vi "[EIP型数字化反应性仪ETH].vi"() -> ()   [LabVIEW 2020]
doc: "该范例演示了通过VI查看其它VI的方法，还可运行和中止查看的VI。\n对于要中止的VI，应设置为可中止。对于无法中止的VI，可查看相关范例。"
uses:
  <vilib>/Utility/error.llb/DialogType.ctl
  GlobalVariable.vi
  TCPModbus_MasterClient/MB Ethernet Master Query Write Multiple Registers (poly).vi
  TCPModbus_MasterClient/MB Ethernet Master Query Read Input Registers (poly).vi
  <vilib>/Analysis/polynomials.llb/Scalar Polynomial Evaluation (DBL).vi
  <vilib>/Analysis/NI_AALPro.lvlib
panel:
  out "上段":bool
  out "下段":bool
  in  "修正因子文件状态":bool
  in  "周期拟合与反应性":bool
  in  "多通道并行实测":bool
  in  "物理参数设置":bool
  in  "打开文件夹":bool
  in  "返回LOGO":bool
  out "项名称":string
  out "退出":bool
  out "MainPanel":enum32{"panel", "logo"}(tab)=enum."logo"
  in  "校准时间":bool
  in  "更新物理参数":bool
  in  "高压2":dbl(slide) scale=-500.0..500.0
  in  "高压1":dbl(slide) scale=-500.0..500.0
  out "P2_8":dbl format="%#.4g"
  out "P2_7":dbl format="%#.4g"
  out "P2_6":dbl format="%#.4g"
  out "P2_5":dbl format="%#.4g"
  out "P2_4":dbl format="%#.4g"
  out "P2_3":dbl format="%#.4g"
  out "P2_1":dbl format="%#.4g"
  in  "离线数据源":bool
  out "电脑历时":dbl format="%#.2g"
  out "程序历时":dbl format="%#.2g"
  out "累计时差":dbl format="%#.4f"
  out "脉冲2":dbl(knob) scale=1.0..1000000.0 scale format="%#_3g"
  out "脉冲3":dbl(knob) scale=1.0..1000000.0 scale format="%#_3g"
  out "电流1":dbl(slide) scale=1e-13..0.0001 scale format="%#_2e"
  out "电流2":dbl(slide) scale=1e-13..0.0001 scale format="%#_2e"
  out "电压1":dbl(knob) scale=1.0..5.0 scale format="%#.4f"
  out "电压2":dbl(knob) scale=1.0..5.0 scale format="%#.4f"
  out "电压3":dbl(knob) scale=1.0..5.0 scale format="%#.4f"
  out "电压4":dbl(knob) scale=1.0..5.0 scale format="%#.4f"
  out "电压5":dbl(knob) scale=1.0..5.0 scale format="%#.4f"
  out "电压6":dbl(knob) scale=1.0..5.0 scale format="%#.4f"
  out "电压7":dbl(knob) scale=1.0..5.0 scale format="%#.4f"
  out "电压8":dbl(knob) scale=1.0..5.0 scale format="%#.4f"
  out "脉冲1":dbl(knob) scale=1.0..1000000.0 scale format="%#_3g"
  out "P2_2":dbl format="%#.4g"
  # "Current1"
  # "Current2"
  # "NetWork"
  # "Voltage Output"
  # "Voltage Input"
  # "AC220V"
  # "Pulse2"
  # "Pulse3"
  # "GND"
  # "Pulse1"
  # "HV1"
  # "HV2"
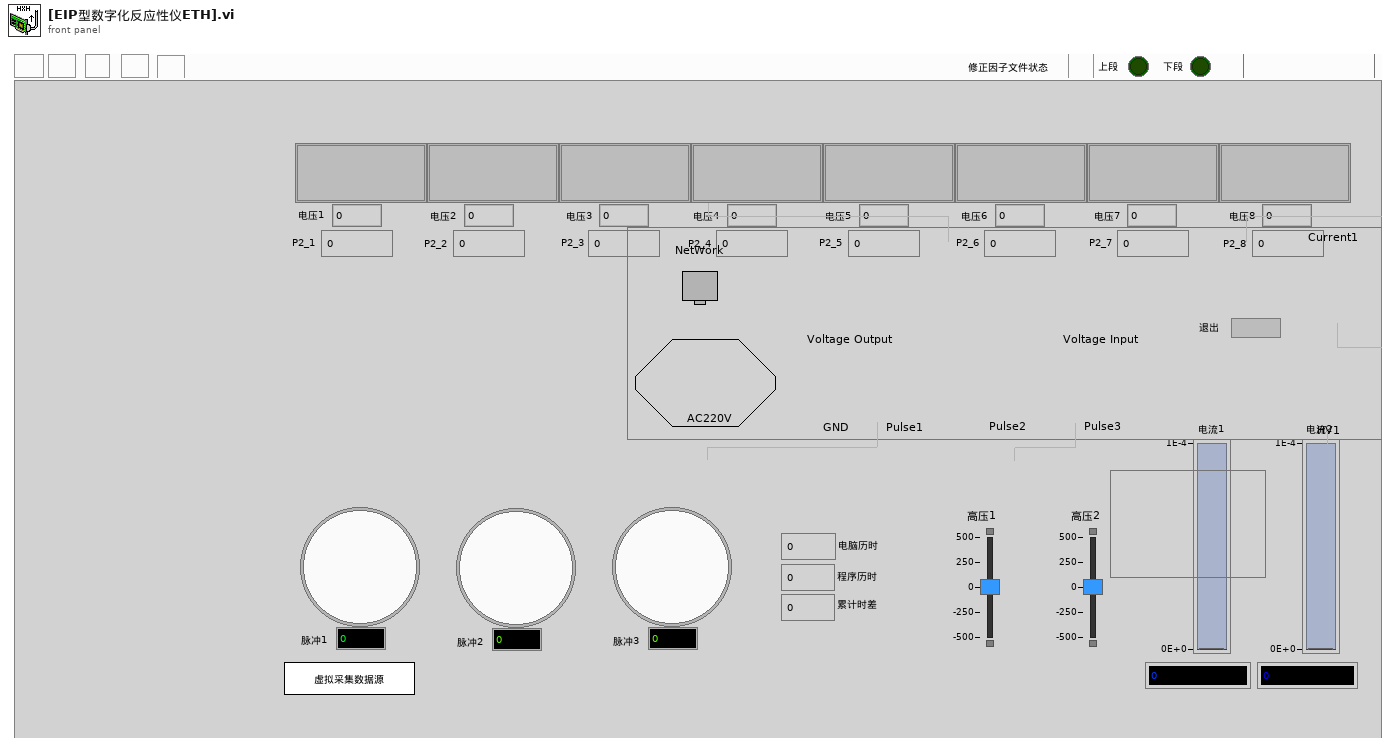
[diagram p1: front panel]
types:
  T1 = typedef "DialogType.ctl" = u16
  T2 = enum32{"Invalid", "Standard", "Closed", "Hidden", "Minimized", "Maximized"}
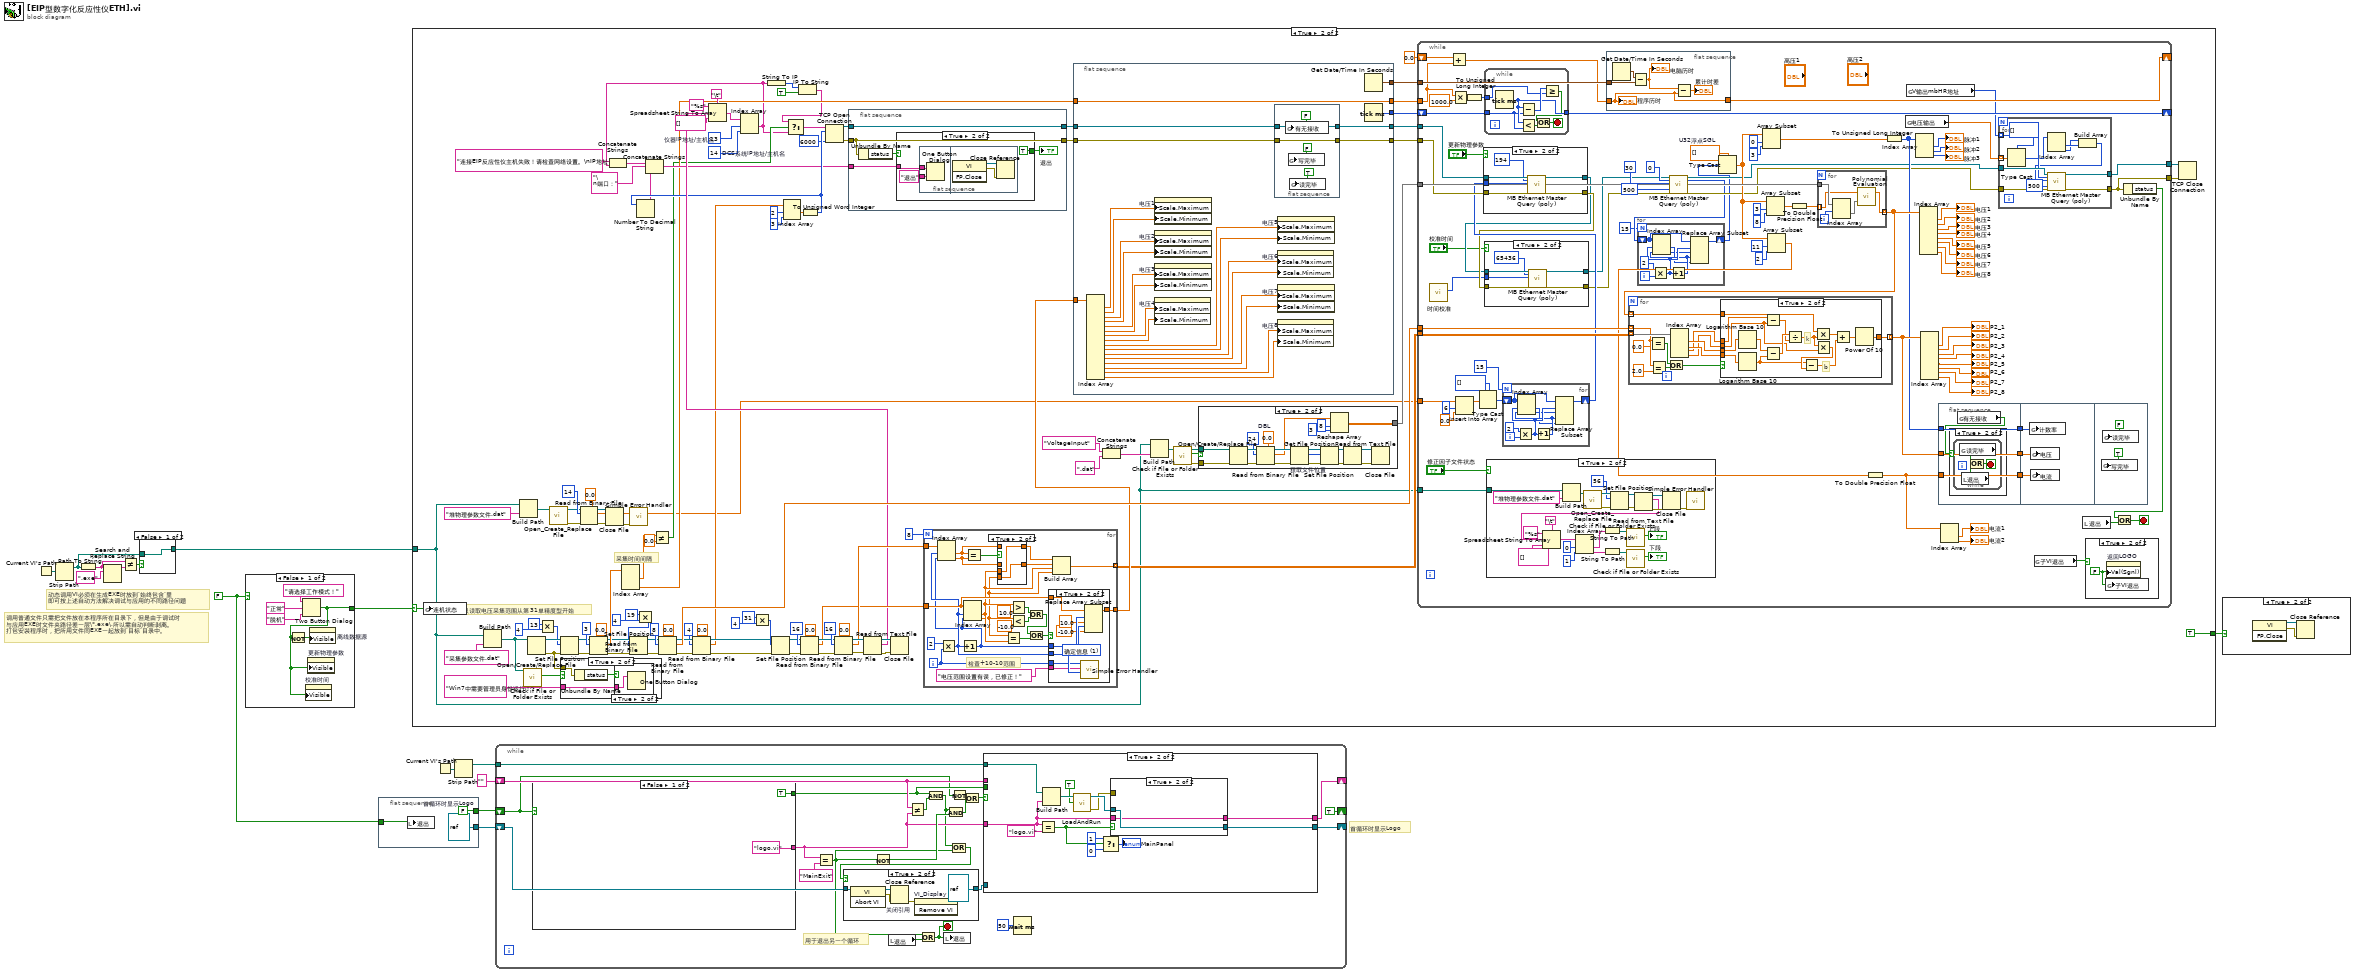
[diagram p0: block diagram]
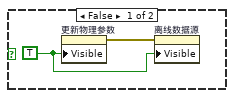
[diagram p2: hidden frame]
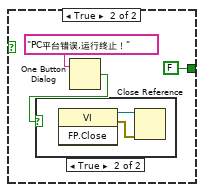
[diagram p3: hidden frame]
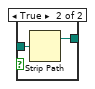
[diagram p5: hidden frame]
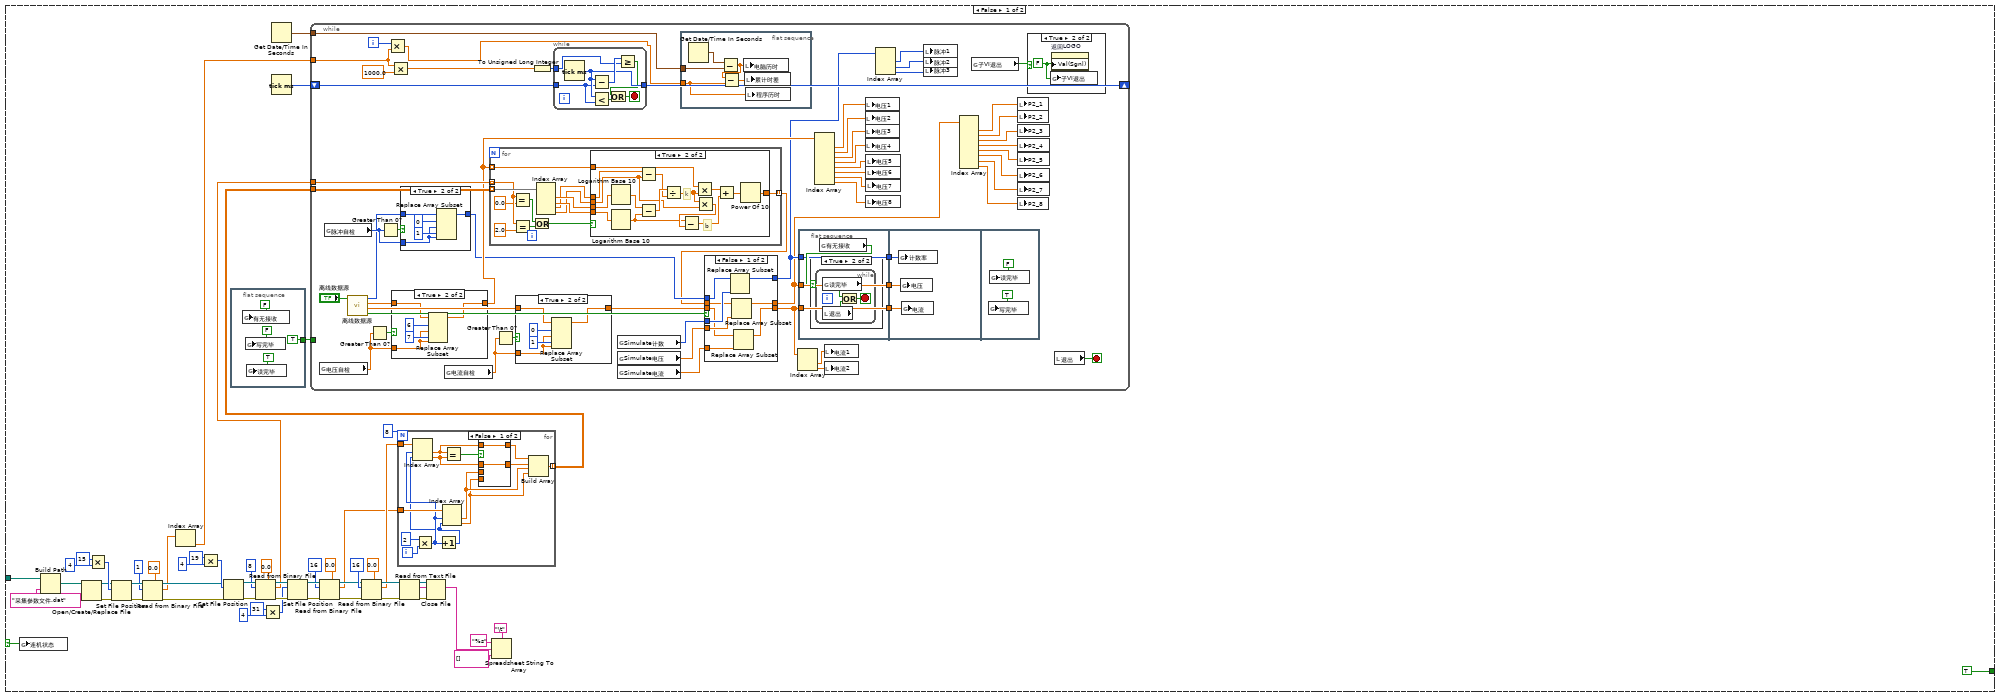
[diagram p6: hidden frame]
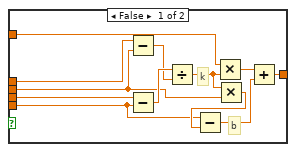
[diagram p12: hidden frame]
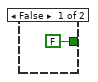
[diagram p15: hidden frame]
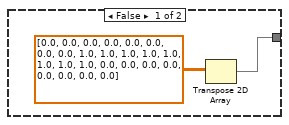
[diagram p18: hidden frame]
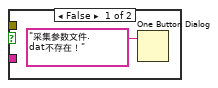
[diagram p19: hidden frame]
diagram:
  w1 = FALSE
  # "调用普通文件只需把文件放在本程序所在目录下，但是由于调试时\n与应用EXE时文件夹路径差一层\\*.exe\\,所以需自动判断剥离。\n打包安装程序时，把所用文件同EXE一起放到‘目标’目录中。"
  # "动态调用VI必须在生成EXE时放到‘始终包含’里\n即可按上述自动方法解决调试与应用的不同路径问题"
  # "首循环时显示Logo"
  n1 = Current VI's Path() -> (path=w10:path)
  n2 = Strip Path(path=w10) -> (stripped path=w5:path)  [unwired: 1 out]
  n3 = Path To String(path=w5) -> (string=w7:string)
  n4 = Search and Replace String(input string=w7, search string=".exe" ("搜索字符串")) -> (result string=w8:string)  [unwired: 6 in, 3 out]
  n5 = Not Equal?(x=w7, y=w8) -> (x != y?=w6:bool)
  n6 = case shown="False" w6 {
    tunnel: w5 -> [w16 w18]
    tunnel: [w16 w17] -> w2
    frame False {
    }
    frame True {
      n7 = Strip Path(path=w18) -> (stripped path=w17:path)  [unwired: 1 out]
    }
  }
  n8 = case shown="False" w1 {
    tunnel: [w19 FALSE ("T button?")] -> w4
    frame False {
      n9 = Two Button Dialog(message="请选择工作模式！" ("消息"), 1:"脱机" ("F按钮名称（“取消”）"), 2:"正常" ("T按钮名称（“确定”）")) -> (T button?=w19:bool)
      n10 = Not(x=w19) -> (.not. x?=w20:bool)
      n11 = property on="校准时间" class="Bool"("Visible"=w19) -> ()  [unwired: 2 in, 2 out]
      n12 = property on="更新物理参数" class="Bool"("Visible"=w19) -> ()  [unwired: 2 in, 2 out]
      n13 = property on="离线数据源" class="Bool"("Visible"=w20) -> ()  [unwired: 2 in, 2 out]
    }
    frame True {
      n14 = One Button Dialog(message="PC平台错误,运行终止！" ("消息")) -> (true=w24:bool)  [unwired: 1 in]
      n15 = case shown="True" w24 {
        frame False {
        }
        frame True {
          n16 = invoke class="VI" method="FP.Close"() -> (reference out=w27:refnum<vi>, error out=w28:errorcluster)  [unwired: 3 in, 1 out]
          n17 = Close Reference(reference=w27, error in (no error)=w28) -> ()  [unwired: 1 out]
        }
      }
    }
  }
  n18 = flat-sequence {
    tunnel: [refnum<vi> refnum ("VI Ref")] -> w15
    tunnel: [w30] -> w14
    tunnel: w1 -> [w29]
    frame #0 {
      w30 = FALSE  # 首循环时显示Logo
      n19 = local write "退出"(w29) -> ()
    }
  }
  n20 = case shown="True" w4 {
    selector: w4 -> [w34 w272]
    tunnel: w2 -> [w64 w266]
    tunnel: [TRUE ("首循环时显示Logo") TRUE ("首循环时显示Logo")] -> w3
    frame False {
      n21 = global write "GlobalVariable.vi" "连机状态"(w34) -> ()
      n22 = Build Path(base path=w64, name or relative path="采集参数文件.dat") -> (appended path=w66:path)
      n23 = Open/Create/Replace File(file path (use dialog)=w66) -> (refnum out=w54:refnum<file>, error out=w53:errorcluster)  [unwired: 5 in, 1 out]
      n24 = Multiply(x=i64 15 ("偏移量（字节）（0）"), y=i64 4 ("偏移量（字节）（0）")) -> (x*y=w61:i64)
      n25 = Set File Position(offset (in bytes) (0)=w61, refnum=w54, error in=w53) -> (refnum out=w57:refnum<file>, error out=w58:errorcluster)  [unwired: 1 in]
      n26 = Read from Binary File(5:sgl 0.0 ("byte stream type"), 8:w58, 10:1 ("count"), 11:w57) -> (0:w51:errorcluster, 2:w50:sgl[], 3:w52:refnum<file>)  [unwired: 2 in, 1 out]
      n27 = Index Array(array=w50) -> (element=w49:sgl)  [unwired: 1 in]
      n28 = Multiply(x=i64 19 ("偏移量（字节）（0）"), y=i64 4 ("偏移量（字节）（0）")) -> (x*y=w73:i64)
      n29 = Set File Position(offset (in bytes) (0)=w73, refnum=w52, error in=w51) -> (refnum out=w69:refnum<file>, error out=w70:errorcluster)  [unwired: 1 in]
      n30 = flat-sequence {
        tunnel: [TRUE ("读完毕")] -> w85
        frame #0 {
          n31 = global write "GlobalVariable.vi" "有无接收"(FALSE ("读完毕")) -> ()
          n32 = global write "GlobalVariable.vi" "写完毕"(FALSE ("读完毕")) -> ()
          n33 = global write "GlobalVariable.vi" "读完毕"(TRUE ("读完毕")) -> ()
        }
      }
      n34 = Read from Binary File(5:sgl 0.0 ("byte stream type"), 8:w70, 10:8 ("count"), 11:w69) -> (0:w81:errorcluster, 2:w63:sgl[], 3:w80:refnum<file>)  [unwired: 2 in, 1 out]
      n35 = Multiply(x=i64 31 ("偏移量（字节）（0）"), y=i64 4 ("偏移量（字节）（0）")) -> (x*y=w79:i64)
      n36 = Get Date/Time In Seconds() -> (seconds since 1Jan1904=w33:timestamp)
      n37 = Tick Count (ms)() -> (millisecond timer value=w32:u32)
      n38 = Set File Position(offset (in bytes) (0)=w79, refnum=w80, error in=w81) -> (refnum out=w76:refnum<file>, error out=w77:errorcluster)  [unwired: 1 in]
      n39 = Read from Binary File(5:sgl 0.0 ("byte stream type"), 8:w77, 10:16 ("count"), 11:w76) -> (0:w45:errorcluster, 2:w40:sgl[], 3:w46:refnum<file>)  [unwired: 2 in, 1 out]
      n40 = Read from Binary File(5:sgl 0.0 ("byte stream type"), 8:w45, 10:16 ("count"), 11:w46) -> (0:w43:errorcluster, 2:w41:sgl[], 3:w44:refnum<file>)  [unwired: 2 in, 1 out]
      n41 = for {
        N: 8 -> [_]
        tunnel: w40 -> [w98]
        tunnel: [w87] -> w39 mode=indexing
        tunnel: w41 -> [w86]
        i -> [w97]
        n42 = Multiply(x=2, y=w97) -> (x*y=w95:i32)
        n43 = Increment(x=w95) -> (x+1=w94:i32)
        n44 = Index Array(array=w86, index #1=w95, index #2=w94) -> (element #1=w93:sgl, element #2=w92:sgl)
        n45 = Index Array(array=w98, index #1=w95, index #2=w94) -> (element #1=w89:sgl, element #2=w88:sgl)
        n46 = Equal?(x=w93, y=w92) -> (x = y?=w96:bool)
        n47 = case shown="False" w96 {
          tunnel: w89 -> [_ w103]
          tunnel: w88 -> [_ w102]
          tunnel: [w101 w103] -> w91
          tunnel: w93 -> [w101 _]
          tunnel: w92 -> [w100 _]
          tunnel: [w100 w102] -> w90
          frame False {
          }
          frame True {
          }
        }
        n48 = Build Array(w91, w90, w89, w88) -> (w87:sgl[])
      }
      n49 = while {
        tunnel: w85 -> [_]
        tunnel: w63 -> [w158]
        tunnel: w49 -> [w135]
        tunnel: w39 -> [w159]
        tunnel: w33 -> [w131]
        shift-right: [w129] -> _
        shift-left: w32 -> [w132]
        i -> [w144]
        stop <- w162 stop-if-true
        n50 = global read "GlobalVariable.vi" "电压自检"() -> (w140:dbl)
        n51 = global read "GlobalVariable.vi" "脉冲自检"() -> (w138:i32)
        n52 = call "离线数据源.vi"("显示前面板"="离线数据源") -> ("前面板打开"=w125:bool, "电流"=w122:dbl[], "电压数据"=w123:dbl[], "脉冲数据"=w124:u32[])  [unwired: 7 in]
        n53 = Greater Than 0?(x=w140) -> (x > 0?=w141:bool)
        n54 = Greater Than 0?(x=w138) -> (x > 0?=w137:bool)
        n55 = Multiply(x=w144, y=w135) -> (x*y=w130:sgl)
        n56 = Multiply(x=w135, y=sgl 1000.0) -> (x*y=w133:sgl)
        n57 = case shown="True" w141 {
          tunnel: w123 -> [w196 w201]
          tunnel: [w196 w200] -> w139
          tunnel: w140 -> [_ w197]
          frame False {
          }
          frame True {
            n58 = Replace Array Subset(array=w201, new element #1=w197, index #1=6 ("索引"), new element #2=w197, index #2=7 ("索引")) -> (w200:dbl[])
          }
        }
        n59 = case shown="True" w137 {
          tunnel: w124 -> [w190 w195]
          tunnel: [w190 w194] -> w119
          tunnel: w138 -> [_ w191]
          frame False {
          }
          frame True {
            n60 = Replace Array Subset(array=w195, new element #1=w191, index #1=0 ("索引"), new element #2=w191, index #2=1 ("索引")) -> (w194:u32[])
          }
        }
        n61 = global read "GlobalVariable.vi" "电流自检"() -> (w142:dbl)
        n62 = for {
          tunnel: w139 -> [w219] mode=indexing
          tunnel: [w208] -> w115 mode=indexing
          tunnel: w159 -> [w220] mode=indexing
          tunnel: w158 -> [w218] mode=indexing
          n63 = Equal?(x=w218, y=sgl 0.0) -> (x = y?=w215:bool)
          n64 = Equal?(x=w218, y=sgl 2.0) -> (x = y?=w214:bool)
          n65 = Or(x=w215, y=w214) -> (x .or. y?=w213:bool)
          n66 = Index Array(array=w220) -> (element #1=w212:sgl, element #2=w211:sgl, element #3=w210:sgl, element #4=w209:sgl)  [unwired: 4 in]
          n67 = case shown="True" w213 {
            tunnel: w219 -> [w232 w238]
            tunnel: [w231 w236] -> w208
            tunnel: w210 -> [w224 w241]
            tunnel: w209 -> [w223 w240]
            tunnel: w212 -> [w222 w234]
            tunnel: w211 -> [w221 w239]
            frame False {
              # "b"
              # "k"
              n68 = Subtract(x=w224, y=w223) -> (x-y=w229:sgl)
              n69 = Subtract(x=w222, y=w221) -> (x-y=w230:sgl)
              n70 = Divide(x=w230, y=w229) -> (x/y=w228:sgl)
              n71 = Multiply(x=w232, y=w228) -> (x*y=w226:dbl)
              n72 = Multiply(x=w228, y=w223) -> (x*y=w227:sgl)
              n73 = Subtract(x=w221, y=w227) -> (x-y=w225:sgl)
              n74 = Add(x=w226, y=w225) -> (x+y=w231:dbl)
            }
            frame True {
              # "b"
              # "k"
              n75 = Logarithm Base 10(1:w234) -> (0:w233:sgl)
              n76 = Logarithm Base 10(1:w239) -> (0:w235:sgl)
              n77 = Subtract(x=w241, y=w240) -> (x-y=w246:sgl)
              n78 = Subtract(x=w233, y=w235) -> (x-y=w247:sgl)
              n79 = Divide(x=w247, y=w246) -> (x/y=w245:sgl)
              n80 = Multiply(x=w238, y=w245) -> (x*y=w243:dbl)
              n81 = Multiply(x=w245, y=w240) -> (x*y=w244:sgl)
              n82 = Subtract(x=w235, y=w244) -> (x-y=w242:sgl)
              n83 = Add(x=w243, y=w242) -> (x+y=w237:dbl)
              n84 = Power Of 10(x=w237) -> (10^x=w236:dbl)
            }
          }
        }
        n85 = Greater Than 0?(x=w142) -> (x > 0?=w143:bool)
        n86 = case shown="True" w143 {
          tunnel: w122 -> [w202 w207]
          tunnel: [w202 w206] -> w121
          tunnel: w142 -> [_ w203]
          frame False {
          }
          frame True {
            n87 = Replace Array Subset(array=w207, new element #1=w203, index #1=0 ("索引"), new element #2=w203, index #2=1 ("索引")) -> (w206:dbl[])
          }
        }
        n88 = To Unsigned Long Integer(number=w133) -> (unsigned 32bit integer=w136:u32)
        n89 = while {
          tunnel: w132 -> [w186]
          tunnel: w136 -> [w188]
          tunnel: [w187] -> w129
          stop <- w183 stop-if-true
          n90 = Tick Count (ms)() -> (millisecond timer value=w187:u32)
          n91 = Subtract(x=w187, y=w186) -> (x-y=w189:u32)
          n92 = Less?(x=w187, y=w186) -> (x < y?=w185:bool)
          n93 = Greater Or Equal?(x=w189, y=w188) -> (x >= y?=w184:bool)
          n94 = Or(x=w184, y=w185) -> (x .or. y?=w183:bool)
        }
        n95 = global read "GlobalVariable.vi" "Simulate计数"() -> (w128:u32[])
        n96 = global read "GlobalVariable.vi" "Simulate电压"() -> (w127:dbl[])
        n97 = global read "GlobalVariable.vi" "Simulate电流"() -> (w126:dbl[])
        n98 = flat-sequence {
          tunnel: w131 -> [w181]
          tunnel: w130 -> [w178]
          frame #0 {
            n99 = Get Date/Time In Seconds() -> (seconds since 1Jan1904=w182:timestamp)
            n100 = Subtract(x=w182, y=w181) -> (x-y=w179:dbl)
            n101 = Subtract(x=w179, y=w178) -> (x-y=w180:dbl)
            n102 = local write "电脑历时"(w179) -> ()
            n103 = local write "累计时差"(w180) -> ()
            n104 = local write "程序历时"(w178) -> ()
          }
        }
        n105 = case shown="False" w125 {
          tunnel: w119 -> [w174 w177]
          tunnel: w115 -> [w170 w176]
          tunnel: w121 -> [w166 w175]
          tunnel: [w172 w177] -> w118
          tunnel: [w169 w176] -> w108
          tunnel: [w168 w175] -> w120
          tunnel: w128 -> [w173 _]
          tunnel: w127 -> [w171 _]
          tunnel: w126 -> [w167 _]
          frame False {
            n106 = Replace Array Subset(array=w174, new element=w173) -> (w172:u32[])  [unwired: 1 in]
            n107 = Replace Array Subset(array=w170, new element=w171) -> (w169:dbl[])  [unwired: 1 in]
            n108 = Replace Array Subset(array=w166, new element=w167) -> (w168:dbl[])  [unwired: 1 in]
          }
          frame True {
          }
        }
        n109 = Index Array(array=w120) -> (element #1=w157:dbl, element #2=w156:dbl)  [unwired: 2 in]
        n110 = flat-sequence {
          tunnel: w120 -> [w251]
          tunnel: w108 -> [w252]
          tunnel: [w252] -> w165
          tunnel: [w251] -> w164
          tunnel: [w249] -> w163
          tunnel: w118 -> [w249]
          tunnel: w165 -> [w258]
          tunnel: w164 -> [w257]
          tunnel: w163 -> [w256]
          frame #0 {
            n111 = global read "GlobalVariable.vi" "有无接收"() -> (w250:bool)
            n112 = case shown="True" w250 {
              frame False {
              }
              frame True {
                n113 = while {
                  stop <- w255 stop-if-true
                  n114 = global read "GlobalVariable.vi" "读完毕"() -> (w254:bool)
                  n115 = local read "退出"() -> (w253:bool)
                  n116 = Or(x=w254, y=w253) -> (x .or. y?=w255:bool)
                }
              }
            }
          }
          frame #1 {
            n117 = global write "GlobalVariable.vi" "计数率"(w256) -> ()
            n118 = global write "GlobalVariable.vi" "电压"(w258) -> ()
            n119 = global write "GlobalVariable.vi" "电流"(w257) -> ()
          }
          frame #2 {
            n120 = global write "GlobalVariable.vi" "写完毕"(TRUE ("写完毕")) -> ()
            n121 = global write "GlobalVariable.vi" "读完毕"(FALSE ("写完毕")) -> ()
          }
        }
        n122 = Index Array(array=w139) -> (element #1=w152:dbl, element #2=w151:dbl, element #3=w150:dbl, element #4=w149:dbl, element #5=w148:dbl, element #6=w147:dbl, element #7=w146:dbl, element #8=w145:dbl)  [unwired: 8 in]
        n123 = local write "电流1"(w157) -> ()
        n124 = local write "电流2"(w156) -> ()
        n125 = local write "电压1"(w152) -> ()
        n126 = local write "电压2"(w151) -> ()
        n127 = local write "电压3"(w150) -> ()
        n128 = local write "电压4"(w149) -> ()
        n129 = local write "电压5"(w148) -> ()
        n130 = local write "电压6"(w147) -> ()
        n131 = local write "电压7"(w146) -> ()
        n132 = local write "电压8"(w145) -> ()
        n133 = Index Array(array=w118) -> (element #1=w155:u32, element #2=w154:u32, element #3=w153:u32)  [unwired: 3 in]
        n134 = local write "脉冲1"(w155) -> ()
        n135 = local write "脉冲2"(w154) -> ()
        n136 = local write "脉冲3"(w153) -> ()
        n137 = Index Array(array=w108) -> (element #1=w117:dbl, element #2=w116:dbl, element #3=w114:dbl, element #4=w113:dbl, element #5=w112:dbl, element #6=w111:dbl, element #7=w110:dbl, element #8=w109:dbl)  [unwired: 8 in]
        n138 = global read "GlobalVariable.vi" "子VI退出"() -> (w160:bool)
        n139 = local write "P2_1"(w117) -> ()
        n140 = local write "P2_2"(w116) -> ()
        n141 = local write "P2_8"(w109) -> ()
        n142 = local write "P2_3"(w114) -> ()
        n143 = local write "P2_4"(w113) -> ()
        n144 = local write "P2_5"(w112) -> ()
        n145 = local write "P2_6"(w111) -> ()
        n146 = local write "P2_7"(w110) -> ()
        n147 = case shown="True" w160 {
          frame False {
          }
          frame True {
            w248 = FALSE ("值(信号)")
            n148 = global write "GlobalVariable.vi" "子VI退出"(w248) -> ()
            n149 = property on="返回LOGO" class="Bool (strict)"("Val(Sgnl)"=w248) -> ()  [unwired: 2 in, 2 out]
          }
        }
        n150 = local read "退出"() -> (w162:bool)
      }
      n151 = Read from Text File(file (use dialog)=w44, error in=w43) -> (refnum out=w83:refnum<file>, text=w35:string, error out=w82:errorcluster)  [unwired: 1 in, 2 out]
      n152 = Close File(refnum=w83, error in=w82) -> ()  [unwired: 2 out]
      n153 = Spreadsheet String To Array(delimiter (Tab)="\t", format string="%s", spreadsheet string=w35, array type (2D Dbl)=string[] [] ("添加的数组")) -> ()  [unwired: 1 out]
    }
    frame True {
      w299 = 14  # DCS系统IP地址/主机名
      w300 = 13  # 仪器IP地址/主机名
      # "采集时间间隔"
      # "只读取电压采集范围从第31单精度型开始"
      n154 = global write "GlobalVariable.vi" "连机状态"(w272) -> ()
      n155 = Build Path(base path=w266, name or relative path="采集参数文件.dat") -> (appended path=w347:path)
      n156 = Build Path(base path=w266, name or relative path="堆物理参数文件.dat" ("string")) -> (appended path=w268:path)
      n157 = call <vilib>:"Check if File or Folder Exists.vi"("path"=w347) -> ("file or folder exists?"=w346:bool)  [unwired: 8 in, 2 out]
      n158 = Open/Create/Replace File(file path (use dialog)=w347) -> (refnum out=w355:refnum<file>, error out=w345:errorcluster)  [unwired: 5 in, 1 out]
      n159 = Multiply(x=i64 13 ("偏移量（字节）（0）"), y=i64 4 ("偏移量（字节）（0）")) -> (x*y=w352:i64)
      n160 = call <vilib>:"Open_Create_Replace File.vi"("file path"=w268) -> ("error out"=w262:errorcluster, "refnum"=w263:refnum<file>)  [unwired: 7 in, 2 out]
      n161 = Set File Position(offset (in bytes) (0)=w352, refnum=w355, error in=w345) -> (refnum out=w357:refnum<file>, error out=w356:errorcluster)  [unwired: 1 in]
      n162 = case shown="True" w346 {
        tunnel: w345 -> [_ w445]
        tunnel: "Win7中需要管理员身份运行！" -> [_ w443]
        frame False {
          n163 = One Button Dialog(message="采集参数文件.dat不存在！" ("消息")) -> ()  [unwired: 1 in, 1 out]
        }
        frame True {
          n164 = Unbundle By Name(w445) -> ("status"=w444:bool)
          n165 = case shown="True" w444 {
            tunnel: w443 -> [_ w446]
            frame False {
            }
            frame True {
              n166 = One Button Dialog(message=w446) -> ()  [unwired: 1 in, 1 out]
            }
          }
        }
      }
      n167 = Read from Binary File(5:sgl 0.0, 8:w262, 10:14, 11:w263) -> (0:w264:errorcluster, 2:w261:sgl[], 3:w265:refnum<file>)  [unwired: 2 in, 1 out]
      n168 = Read from Binary File(5:sgl 0.0 ("byte stream type"), 8:w356, 10:3 ("count"), 11:w357) -> (0:w338:errorcluster, 2:w350:sgl[], 3:w339:refnum<file>)  [unwired: 2 in, 1 out]
      n169 = Close File(refnum=w265, error in=w264) -> (error out=w267:errorcluster)  [unwired: 1 out]
      n170 = Index Array(array=w350) -> (element #1=w280:sgl, element #3=w282:sgl)  [unwired: 3 in, 1 out]
      n171 = call <vilib>:"Simple Error Handler.vi"("error in (no error)"=w267) -> ()  [unwired: 4 in, 5 out]
      n172 = Multiply(x=i64 19 ("偏移量（字节）（0）"), y=i64 4 ("偏移量（字节）（0）")) -> (x*y=w335:i64)
      n173 = Set File Position(offset (in bytes) (0)=w335, refnum=w339, error in=w338) -> (refnum out=w341:refnum<file>, error out=w340:errorcluster)  [unwired: 1 in]
      n174 = Not Equal?(x=w280, y=sgl 0.0) -> (x != y?=w278:bool)
      n175 = Read from Binary File(5:sgl 0.0 ("byte stream type"), 8:w340, 10:8 ("count"), 11:w341) -> (0:w297:errorcluster, 2:w334:sgl[], 3:w296:refnum<file>)  [unwired: 2 in, 1 out]
      n176 = Read from Binary File(5:sgl 0.0 ("byte stream type"), 8:w297, 10:4 ("count"), 11:w296) -> (0:w294:errorcluster, 2:w292:sgl[], 3:w295:refnum<file>)  [unwired: 2 in, 1 out]
      n177 = Multiply(x=i64 31 ("偏移量（字节）（0）"), y=i64 4 ("偏移量（字节）（0）")) -> (x*y=w360:i64)
      n178 = Set File Position(offset (in bytes) (0)=w360, refnum=w295, error in=w294) -> (refnum out=w366:refnum<file>, error out=w365:errorcluster)  [unwired: 1 in]
      n179 = Index Array(array=w292, index #1=2 ("索引"), index #2=3 ("索引")) -> (element #1=w291:sgl)  [unwired: 1 out]
      n180 = Read from Binary File(5:sgl 0.0 ("byte stream type"), 8:w365, 10:16 ("count"), 11:w366) -> (0:w324:errorcluster, 2:w320:sgl[], 3:w325:refnum<file>)  [unwired: 2 in, 1 out]
      n181 = To Unsigned Word Integer(number=w291) -> (unsigned 16bit integer=w288:u16)
      n182 = Number To Decimal String(number=w288) -> (decimal integer string=w287:string)  [unwired: 1 in]
      n183 = Read from Binary File(5:sgl 0.0 ("byte stream type"), 8:w324, 10:16 ("count"), 11:w325) -> (0:w322:errorcluster, 2:w321:sgl[], 3:w323:refnum<file>)  [unwired: 2 in, 1 out]
      n184 = flat-sequence {
        tunnel: w311 -> [w375]
        tunnel: w310 -> [w374]
        tunnel: [w375] -> w309
        tunnel: [w374] -> w308
        tunnel: w285 -> [w371]
        frame #0 {
          n185 = Unbundle By Name(w374) -> ("status"=w373:bool)
          n186 = case shown="True" w373 {
            tunnel: [FALSE ("退出") TRUE ("退出")] -> w372
            tunnel: w371 -> [_ w378]
            frame False {
            }
            frame True {
              n187 = flat-sequence {
                tunnel: w378 -> [w381]
                tunnel: "退出" ("按钮名称（“确定”）") -> [w380]
                frame #0 {
                  n188 = One Button Dialog(message=w381, button name ("OK")=w380) -> ()  [unwired: 1 out]
                }
                frame #1 {
                  n189 = invoke class="VI" method="FP.Close"() -> (reference out=w382:refnum<vi>, error out=w383:errorcluster)  [unwired: 3 in, 1 out]
                  n190 = Close Reference(reference=w382, error in (no error)=w383) -> ()  [unwired: 1 out]
                }
              }
            }
          }
          "退出" <- w372
        }
      }
      n191 = Read from Text File(file (use dialog)=w323, error in=w322) -> (refnum out=w363:refnum<file>, text=w302:string, error out=w364:errorcluster)  [unwired: 1 in, 2 out]
      n192 = Spreadsheet String To Array(delimiter (Tab)="\t", format string="%s", spreadsheet string=w302, array type (2D Dbl)=string[] [] ("添加的数组")) -> (array=w301:string[])
      n193 = Index Array(array=w301, index #1=w300, index #2=w299) -> (element #1=w277:string)  [unwired: 1 out]
      n194 = Concatenate Strings("连接EIP反应性仪主机失败！请检查网络设置。\nIP地址：" ("消息"), w277) -> (w289:string)
      n195 = Concatenate Strings(w289, "\n端口：" ("字符串"), w287) -> (w285:string)
      n196 = String To IP(1:w277) -> (0:w275:u32)
      n197 = IP To String(1:TRUE ("句点符号？(F)"), 2:w275) -> (0:w274:string)
      n198 = Select(t=w274, s=w278, f=w277) -> (s? t:f=w279:string)
      n199 = TCP Open Connection(address=w279, remote port or service name=w288, timeout ms (60000)=6000 ("超时毫秒(60000)")) -> (connection ID=w311:refnum<k5>, error out=w310:errorcluster)  [unwired: 1 in, 1 out]
      n200 = Close File(refnum=w363, error in=w364) -> ()  [unwired: 2 out]
      n201 = for {
        N: 8 -> [_]
        tunnel: w320 -> [w401]
        tunnel: [w400] -> w319
        tunnel: [w385] -> w318 mode=indexing
        tunnel: w321 -> [w384]
        i -> [w398]
        # "检查+10-10范围"
        n202 = Multiply(x=2, y=w398) -> (x*y=w396:i32)
        n203 = Increment(x=w396) -> (x+1=w395:i32)
        n204 = Index Array(array=w384, index #1=w396, index #2=w395) -> (element #1=w394:sgl, element #2=w393:sgl)
        n205 = Index Array(array=w401, index #1=w396, index #2=w395) -> (element #1=w387:sgl, element #2=w386:sgl)
        n206 = Equal?(x=w394, y=w393) -> (x = y?=w397:bool)
        n207 = case shown="True" w397 {
          tunnel: w387 -> [_ w410]
          tunnel: w386 -> [_ w409]
          tunnel: [w408 w410] -> w389
          tunnel: w394 -> [w408 _]
          tunnel: w393 -> [w407 _]
          tunnel: [w407 w409] -> w388
          frame False {
          }
          frame True {
          }
        }
        n208 = Equal?(x=w386, y=w387) -> (x = y?=w391:bool)
        n209 = Greater?(x=w387, y=10.0) -> (0:w403:bool)
        n210 = Less?(x=w386, y=sgl -10.0) -> (x < y?=w402:bool)
        n211 = Or(x=w403, y=w402) -> (x .or. y?=w392:bool)
        n212 = Or(x=w392, y=w391) -> (x .or. y?=w390:bool)
        n213 = case shown="True" w390 {
          tunnel: w401 -> [w411 w420]
          tunnel: [w411 w419] -> w400
          tunnel: w395 -> [_ w418]
          tunnel: w396 -> [_ w417]
          tunnel: "电压范围设置有误，已修正！" ("error source (\" \")") -> [_ w413]
          tunnel: w398 -> [_ w412]
          frame False {
          }
          frame True {
            w414 = T1 1 items=["无对话框", "确定信息", "继续或停止信息", "确定信息＋警告", "继续/停止+警告"] ("type of dialog (OK msg:1)")
            n214 = call <vilib>:"Simple Error Handler.vi"("error code (no error:0)"=w412, "error source (\" \")"=w413, "type of dialog (OK msg:1)"=w414) -> ()  [unwired: 2 in, 5 out]
            n215 = Replace Array Subset(array=w420, new element #1=sgl 10.0 ("新元素/子数组"), index #1=w417, new element #2=sgl -10.0 ("新元素/子数组"), index #2=w418) -> (w419:sgl[])
          }
        }
        n216 = Build Array(w389, w388, w387, w386) -> (w385:sgl[])
      }
      n217 = flat-sequence {
        tunnel: [w470] -> w370
        tunnel: w319 -> [w469]
        tunnel: [w452] -> w359
        tunnel: w282 -> [w452]
        tunnel: [w447] -> w315
        tunnel: [w449] -> w314
        tunnel: [w451] -> w313
        tunnel: w309 -> [w448]
        tunnel: w308 -> [w450]
        frame #0 {
          n218 = Index Array(array=w469) -> (element #1=w461:sgl, element #2=w468:sgl, element #3=w460:sgl, element #4=w459:sgl, element #5=w458:sgl, element #6=w467:sgl, element #7=w457:sgl, element #8=w466:sgl, element #9=w456:sgl, element #10=w465:sgl, element #11=w455:sgl, element #12=w464:sgl, element #13=w454:sgl, element #14=w463:sgl, element #15=w453:sgl, element #16=w462:sgl)  [unwired: 16 in]
          n219 = property on="电压4" class="Knob (strict)"("Scale.Maximum"=w457, "Scale.Minimum"=w466) -> ()  [unwired: 2 in, 2 out]
          n220 = property on="电压1" class="Knob (strict)"("Scale.Maximum"=w461, "Scale.Minimum"=w468) -> ()  [unwired: 2 in, 2 out]
          n221 = property on="电压2" class="Knob (strict)"("Scale.Maximum"=w460, "Scale.Minimum"=w459) -> ()  [unwired: 2 in, 2 out]
          n222 = property on="电压3" class="Knob (strict)"("Scale.Maximum"=w458, "Scale.Minimum"=w467) -> ()  [unwired: 2 in, 2 out]
          n223 = flat-sequence {
            tunnel: w450 -> [w472]
            tunnel: [w472] -> w449
            tunnel: w448 -> [w471]
            tunnel: [w471] -> w447
            frame #0 {
              n224 = global write "GlobalVariable.vi" "有无接收"(FALSE ("读完毕")) -> ()
              n225 = global write "GlobalVariable.vi" "写完毕"(FALSE ("读完毕")) -> ()
              n226 = global write "GlobalVariable.vi" "读完毕"(TRUE ("读完毕")) -> ()
            }
          }
          n227 = property on="电压6" class="Knob (strict)"("Scale.Maximum"=w455, "Scale.Minimum"=w464) -> ()  [unwired: 2 in, 2 out]
          n228 = property on="电压8" class="Knob (strict)"("Scale.Maximum"=w453, "Scale.Minimum"=w462) -> ()  [unwired: 2 in, 2 out]
          n229 = property on="电压5" class="Knob (strict)"("Scale.Maximum"=w456, "Scale.Minimum"=w465) -> ()  [unwired: 2 in, 2 out]
          n230 = property on="电压7" class="Knob (strict)"("Scale.Maximum"=w454, "Scale.Minimum"=w463) -> ()  [unwired: 2 in, 2 out]
          n231 = Get Date/Time In Seconds() -> (seconds since 1Jan1904=w470:timestamp)
          n232 = Tick Count (ms)() -> (millisecond timer value=w451:u32)
        }
      }
      n233 = Concatenate Strings("VoltageInput", ".dat") -> (w328:string)
      n234 = Build Path(base path=w266, name or relative path=w328) -> (appended path=w333:path)
      n235 = call <vilib>:"Check if File or Folder Exists.vi"("path"=w333) -> ("error out"=w331:errorcluster, "file or folder exists?"=w330:bool, "dup path"=w332:path)  [unwired: 8 in]
      n236 = case shown="True" w330 {
        tunnel: [w421 w425] -> w348
        tunnel: w332 -> [_ w424]
        tunnel: w331 -> [_ w423]
        frame False {
          n237 = Transpose 2D Array(2D array=dbl[][] [[0.0, 0.0, 0.0, 0.0, 0.0, 0.0, 0.0, 0.0], [1.0, 1.0, 1.0, 1.0, 1.0, 1.0, 1.0, 1.0], [0.0, 0.0, 0.0, 0.0, 0.0, 0.0, 0.0, 0.0]]) -> (transposed array=w421:dbl[][])
        }
        frame True {
          w438 = 0.0  # DBL
          n238 = Open/Create/Replace File(file path (use dialog)=w424, error in=w423) -> (refnum out=w441:refnum<file>, error out=w440:errorcluster)  [unwired: 4 in, 1 out]
          n239 = Read from Binary File(5:w438, 8:w440, 10:24 ("count"), 11:w441) -> (0:w429:errorcluster, 2:w426:dbl[], 3:w430:refnum<file>)  [unwired: 2 in, 1 out]
          n240 = Get File Position "获取文件位置"(4:w429, 7:w430) -> (0:w436:errorcluster, 2:w435:i64, 3:w437:refnum<file>)
          n241 = Set File Position(offset (in bytes) (0)=w435, refnum=w437, error in=w436) -> (refnum out=w434:refnum<file>, error out=w433:errorcluster)  [unwired: 1 in]
          n242 = Reshape Array(w426, 8 ("维数大小"), 3 ("维数大小")) -> (w425:dbl[][])
          n243 = Read from Text File(file (use dialog)=w434, error in=w433) -> (refnum out=w432:refnum<file>, error out=w431:errorcluster)  [unwired: 1 in, 3 out]
          n244 = Close File(refnum=w432, error in=w431) -> ()  [unwired: 2 out]
        }
      }
      n245 = while {
        tunnel: w359 -> [w513]
        tunnel: w370 -> [w560]
        tunnel: w348 -> [w559]
        tunnel: w334 -> [w557]
        tunnel: w318 -> [w556]
        tunnel: w315 -> [w499]
        tunnel: w314 -> [w498]
        shift-right: [w515] -> _
        shift-left: w313 -> [w519]
        shift-right: [w511] -> _
        shift-left: sgl 0.0 ("byte stream type") -> [w514]
        tunnel: [w504] -> w307
        tunnel: [w505] -> w306
        tunnel: w266 -> [w501]
        tunnel: w261 -> [w490]
        stop <- w510 stop-if-true
        w487 = sgl[] []  # U32浮点SGL
        n246 = call "时间校准.vi"() -> ("DTout"=w477:u16[])  [unwired: 11 in]
        n247 = Add(x=w514, y=w513) -> (x+y=w512:sgl)
        n248 = Multiply(x=w513, y=sgl 1000.0) -> (x*y=w517:sgl)
        n249 = Insert Into Array(array=w490, index=6 ("索引"), new element=sgl 0.0 ("新元素/子数组")) -> (w491:sgl[])
        n250 = To Unsigned Long Integer(number=w517) -> (unsigned 32bit integer=w516:u32)
        n251 = Type Cast(type=u16[] [] ("Input Registers"), x=w491) -> (*(type *) &x=w495:u16[])
        n252 = while {
          tunnel: w519 -> [w635]
          tunnel: w516 -> [w637]
          tunnel: [w636] -> w515
          stop <- w632 stop-if-true
          n253 = Tick Count (ms)() -> (millisecond timer value=w636:u32)
          n254 = Subtract(x=w636, y=w635) -> (x-y=w638:u32)
          n255 = Less?(x=w636, y=w635) -> (x < y?=w634:bool)
          n256 = Greater Or Equal?(x=w638, y=w637) -> (x >= y?=w633:bool)
          n257 = Or(x=w633, y=w634) -> (x .or. y?=w632:bool)
        }
        n258 = case shown="True" "修正因子文件状态" {
          tunnel: w501 -> [_ w600]
          frame False {
          }
          frame True {
            n259 = Build Path(base path=w600, name or relative path="堆物理参数文件.dat" ("string")) -> (appended path=w618:path)
            n260 = call <vilib>:"Open_Create_Replace File.vi"("file path"=w618) -> ("error out"=w616:errorcluster, "refnum"=w617:refnum<file>)  [unwired: 7 in, 2 out]
            n261 = Set File Position(offset (in bytes) (0)=i64 56 ("偏移量（字节）（0）"), refnum=w617, error in=w616) -> (refnum out=w606:refnum<file>, error out=w605:errorcluster)  [unwired: 1 in]
            n262 = Read from Text File(file (use dialog)=w606, error in=w605) -> (refnum out=w603:refnum<file>, text=w601:string, error out=w602:errorcluster)  [unwired: 1 in, 2 out]
            n263 = Spreadsheet String To Array(delimiter (Tab)="\t", format string="%s", spreadsheet string=w601, array type (2D Dbl)=string[] [] ("添加的数组")) -> (array=w609:string[])
            n264 = Index Array(array=w609, index #1=0 ("index"), index #2=1 ("index")) -> (element #1=w608:string, element #2=w598:string)
            n265 = String To Path(string=w608) -> (path=w607:path)
            n266 = String To Path(string=w598) -> (path=w599:path)
            n267 = call <vilib>:"Check if File or Folder Exists.vi"("path"=w607) -> ("file or folder exists?"=→"上段":bool)  [unwired: 8 in, 2 out]
            n268 = call <vilib>:"Check if File or Folder Exists.vi"("path"=w599) -> ("file or folder exists?"=→"下段":bool)  [unwired: 8 in, 2 out]
            n269 = Close File(refnum=w603, error in=w602) -> (error out=w604:errorcluster)  [unwired: 1 out]
            n270 = call <vilib>:"Simple Error Handler.vi"("error in (no error)"=w604) -> ()  [unwired: 4 in, 5 out]
          }
        }
        n271 = for {
          N: 15 -> [_]
          shift-right: [w580] -> w489
          shift-left: w495 -> [w585]
          i -> [w587]
          n272 = Multiply(x=2, y=w587) -> (x*y=w584:i32)
          n273 = Increment(x=w584) -> (x+1=w583:i32)
          n274 = Index Array(array=w585, index #1=w584, index #2=w583) -> (element #1=w582:u16, element #2=w581:u16)
          n275 = Replace Array Subset(array=w585, new element #1=w581, index #1=w584, new element #2=w582, index #2=w583) -> (w580:u16[])
        }
        n276 = case shown="True" "更新物理参数" {
          tunnel: w499 -> [w589 w595]
          tunnel: w498 -> [w588 w594]
          tunnel: [w589 w593] -> w481
          tunnel: [w588 w592] -> w482
          tunnel: w489 -> [_ w590]
          frame False {
          }
          frame True {
            n277 = call-poly "MB Ethernet Master Query (poly).vi"("TCP Connection Refnum in"=w595, "Starting Address"=u16 194, "Registers"=w590, "error in"=w594) -> ("TCP Connection Refnum (dup)"=w593:refnum<k5>, "error out"=w592:errorcluster)  [unwired: 2 in, 12 out]
          }
        }
        n278 = case shown="True" "校准时间" {
          tunnel: w481 -> [w565 w571]
          tunnel: w482 -> [w564 w570]
          tunnel: [w565 w569] -> w480
          tunnel: [w564 w568] -> w479
          tunnel: w477 -> [_ w566]
          frame False {
          }
          frame True {
            n279 = call-poly "MB Ethernet Master Query (poly).vi"("TCP Connection Refnum in"=w571, "Starting Address"=u16 65436, "Registers"=w566, "error in"=w570) -> ("TCP Connection Refnum (dup)"=w569:refnum<k5>, "error out"=w568:errorcluster)  [unwired: 2 in, 12 out]
          }
        }
        n280 = flat-sequence {
          tunnel: w512 -> [w697]
          tunnel: w560 -> [w698]
          tunnel: [w697] -> w511
          frame #0 {
            n281 = Get Date/Time In Seconds() -> (seconds since 1Jan1904=w699:timestamp)
            n282 = Subtract(x=w699, y=w698) -> (x-y=w700:dbl)
            "电脑历时" <- w700
            n283 = Subtract(x=w700, y=w697) -> (x-y=→"累计时差":dbl)
            "程序历时" <- w697
          }
        }
        n284 = call-poly "MB Ethernet Master Query (poly).vi"("TCP Connection Refnum in"=w480, "Starting Address"=u16 0, "Quantity"=u16 30 ("modbus寄存器数量"), "Timeout"=500, "error in"=w479) -> ("TCP Connection Refnum (dup)"=w506:refnum<k5>, "Input Registers"=w485:u16[], "error out"=w507:errorcluster)  [unwired: 12 out]
        n285 = for {
          N: 15 -> [_]
          shift-right: [w572] -> w484
          shift-left: w485 -> [w577]
          i -> [w579]
          n286 = Multiply(x=2, y=w579) -> (x*y=w576:i32)
          n287 = Increment(x=w576) -> (x+1=w575:i32)
          n288 = Index Array(array=w577, index #1=w576, index #2=w575) -> (element #1=w574:u16, element #2=w573:u16)
          n289 = Replace Array Subset(array=w577, new element #1=w573, index #1=w576, new element #2=w574, index #2=w575) -> (w572:u16[])
        }
        n290 = Type Cast(type=w487, x=w484) -> (*(type *) &x=w522:sgl[])
        n291 = Array Subset(array=w522, index=0 ("索引"), length=3 ("长度")) -> (w528:sgl[])
        n292 = Array Subset(array=w522, index=3 ("索引"), length=8 ("长度")) -> (w525:sgl[])
        n293 = Array Subset(array=w522, index=11 ("索引"), length=2 ("长度")) -> (w521:sgl[])
        n294 = To Double Precision Float(number=w525) -> (double precision float=w531:dbl[])
        n295 = for {
          tunnel: w531 -> [w640] mode=indexing
          tunnel: [w639] -> w544 mode=indexing
          tunnel: w559 -> [w642]
          i -> [w641]
          n296 = Index Array(array=w642, index (row)=w641) -> (element=w643:dbl[])  [unwired: 1 in]
          n297 = call-poly <vilib>:"Polynomial Evaluation.vi"("P(x)"=w643, "a"=w640) -> ("P(a)"=w639:dbl)  [unwired: 1 out]
        }
        n298 = for {
          tunnel: w544 -> [w655] mode=indexing
          tunnel: [w654] -> w541 mode=indexing
          tunnel: w556 -> [w656] mode=indexing
          tunnel: w557 -> [w653] mode=indexing
          n299 = Equal?(x=w653, y=sgl 0.0) -> (x = y?=w650:bool)
          n300 = Equal?(x=w653, y=sgl 2.0) -> (x = y?=w649:bool)
          n301 = Or(x=w650, y=w649) -> (x .or. y?=w648:bool)
          n302 = Index Array(array=w656) -> (element #1=w647:sgl, element #2=w646:sgl, element #3=w645:sgl, element #4=w644:sgl)  [unwired: 4 in]
          n303 = case shown="True" w648 {
            tunnel: w655 -> [w668 w674]
            tunnel: [w667 w672] -> w654
            tunnel: w645 -> [w660 w677]
            tunnel: w644 -> [w659 w676]
            tunnel: w647 -> [w658 w670]
            tunnel: w646 -> [w657 w675]
            frame False {
              # "b"
              # "k"
              n304 = Subtract(x=w660, y=w659) -> (x-y=w665:sgl)
              n305 = Subtract(x=w658, y=w657) -> (x-y=w666:sgl)
              n306 = Divide(x=w666, y=w665) -> (x/y=w664:sgl)
              n307 = Multiply(x=w668, y=w664) -> (x*y=w662:dbl)
              n308 = Multiply(x=w664, y=w659) -> (x*y=w663:sgl)
              n309 = Subtract(x=w657, y=w663) -> (x-y=w661:sgl)
              n310 = Add(x=w662, y=w661) -> (x+y=w667:dbl)
            }
            frame True {
              # "b"
              # "k"
              n311 = Logarithm Base 10(1:w670) -> (0:w669:sgl)
              n312 = Logarithm Base 10(1:w675) -> (0:w671:sgl)
              n313 = Subtract(x=w677, y=w676) -> (x-y=w682:sgl)
              n314 = Subtract(x=w669, y=w671) -> (x-y=w683:sgl)
              n315 = Divide(x=w683, y=w682) -> (x/y=w681:sgl)
              n316 = Multiply(x=w674, y=w681) -> (x*y=w679:dbl)
              n317 = Multiply(x=w681, y=w676) -> (x*y=w680:sgl)
              n318 = Subtract(x=w671, y=w680) -> (x-y=w678:sgl)
              n319 = Add(x=w679, y=w678) -> (x+y=w673:dbl)
              n320 = Power Of 10(x=w673) -> (10^x=w672:dbl)
            }
          }
        }
        n321 = To Double Precision Float(number=w521) -> (double precision float=w520:dbl[])
        n322 = To Unsigned Long Integer(number=w528) -> (unsigned 32bit integer=w532:u32[])
        n323 = global read "GlobalVariable.vi" "电压输出"() -> (w503:sgl[])
        n324 = global read "GlobalVariable.vi" "V输出mbHR地址"() -> (w502:u16[])
        n325 = Index Array(array=w532) -> (element #1=→"脉冲1":u32, element #2=→"脉冲2":u32, element #3=→"脉冲3":u32)  [unwired: 3 in]
        n326 = Index Array(array=w544) -> (element #1=→"电压1":dbl, element #2=→"电压2":dbl, element #3=→"电压3":dbl, element #4=→"电压4":dbl, element #5=→"电压5":dbl, element #6=→"电压6":dbl, element #7=→"电压7":dbl, element #8=→"电压8":dbl)  [unwired: 8 in]
        n327 = Index Array(array=w541) -> (element #1=→"P2_1":dbl, element #2=→"P2_2":dbl, element #3=→"P2_3":dbl, element #4=→"P2_4":dbl, element #5=→"P2_5":dbl, element #6=→"P2_6":dbl, element #7=→"P2_7":dbl, element #8=→"P2_8":dbl)  [unwired: 8 in]
        n328 = flat-sequence {
          tunnel: w532 -> [w686]
          tunnel: w520 -> [w687]
          tunnel: w541 -> [w688]
          tunnel: [w688] -> w563
          tunnel: [w687] -> w562
          tunnel: [w686] -> w561
          tunnel: w563 -> [w694]
          tunnel: w562 -> [w693]
          tunnel: w561 -> [w692]
          frame #0 {
            n329 = global read "GlobalVariable.vi" "有无接收"() -> (w685:bool)
            n330 = case shown="True" w685 {
              frame False {
              }
              frame True {
                n331 = while {
                  stop <- w690 stop-if-true
                  n332 = global read "GlobalVariable.vi" "读完毕"() -> (w689:bool)
                  n333 = local read "退出"() -> (w691:bool)
                  n334 = Or(x=w689, y=w691) -> (x .or. y?=w690:bool)
                }
              }
            }
          }
          frame #1 {
            n335 = global write "GlobalVariable.vi" "计数率"(w692) -> ()
            n336 = global write "GlobalVariable.vi" "电压"(w694) -> ()
            n337 = global write "GlobalVariable.vi" "电流"(w693) -> ()
          }
          frame #2 {
            n338 = global write "GlobalVariable.vi" "写完毕"(TRUE ("写完毕")) -> ()
            n339 = global write "GlobalVariable.vi" "读完毕"(FALSE ("写完毕")) -> ()
          }
        }
        n340 = Index Array(array=w520) -> (element #1=→"电流1":dbl, element #2=→"电流2":dbl)  [unwired: 2 in]
        n341 = for {
          tunnel: w507 -> [w631]
          tunnel: w506 -> [w630]
          tunnel: [w629] -> w505
          tunnel: [w628] -> w504
          tunnel: w503 -> [w627] mode=indexing
          tunnel: w502 -> [w626] mode=indexing
          n342 = Type Cast(type=u16[] [] ("Input Registers"), x=w627) -> (*(type *) &x=w624:u16[])
          n343 = Index Array(array=w624) -> (element #1=w623:u16, element #2=w622:u16)  [unwired: 2 in]
          n344 = Build Array(w622, w623) -> (w621:u16[])
          n345 = call-poly "MB Ethernet Master Query (poly).vi"("TCP Connection Refnum in"=w630, "Starting Address"=w626, "Registers"=w621, "Timeout"=u32 500, "error in"=w631) -> ("TCP Connection Refnum (dup)"=w628:refnum<k5>, "error out"=w629:errorcluster)  [unwired: 1 in, 12 out]
        }
        n346 = global read "GlobalVariable.vi" "子VI退出"() -> (w558:bool)
        n347 = local read "退出"() -> (w509:bool)
        n348 = case shown="True" w558 {
          frame False {
          }
          frame True {
            w684 = FALSE ("值(信号)")
            n349 = global write "GlobalVariable.vi" "子VI退出"(w684) -> ()
            n350 = property on="返回LOGO" class="Bool (strict)"("Val(Sgnl)"=w684) -> ()  [unwired: 2 in, 2 out]
          }
        }
        n351 = Unbundle By Name(w505) -> ("status"=w508:bool)
        n352 = Or(x=w508, y=w509) -> (x .or. y?=w510:bool)
      }
      n353 = TCP Close Connection ("关闭TCP连接")(connection ID=w307, error in (no error)=w306) -> ()  [unwired: 3 out]
    }
  }
  n354 = Current VI's Path() -> (path=w12:path)
  n355 = Strip Path(path=w12) -> (stripped path=w11:path)  [unwired: 1 out]
  n356 = while {
    shift-right: [w723] -> _
    shift-left: w15 -> [w718]
    shift-right: [w722] -> _
    shift-left: "" ("ItemTag") -> [w709]
    shift-right: [TRUE ("首循环时显示Logo")] -> _
    shift-left: w14 -> [w702]
    tunnel: w11 -> [w719]
    stop <- w720 stop-if-true
    # "用于退出另一个循环"
    n357 = case shown="False" w702 {
      tunnel: ["logo.vi" ("ItemTag") w782] -> w708
      tunnel: [TRUE w775] -> w703
      frame False {
      }
      frame True {
        n358 = event shown="[1] \"返回LOGO\": Value Change" {
          selector: _ -> [_ _ _ _ _ _]
          dyn-events: _ -> [_ _ _ _ _ _]
          timeout: _ -> [_ _ _ _ _ _]
          tunnel: [w793 "logo.vi" ("ItemTag") "打开数据文件夹.vi" ("ItemTag") "堆物理参数设置.vi" ("ItemTag") "多通道并行实测\\多通道并行实测.vi" ("ItemTag") "周期拟合倒时反应性.vi" ("ItemTag")] -> w773
          tunnel: [w792 "仪器设置:" ("ItemPath") "" ("ItemPath") "仪器设置:" ("x") "实时测量:" ("x") "数据处理:" ("x")] -> w774
          event Menu Selection (User) {
            n359 = event-data() -> ("ItemPath"=w792:string, "MenuRef"=w794:refnum<k9>, "ItemTag"=w793:string)  [unwired: 1 out]
            n360 = case shown="Default" w793 {
              tunnel: w793 -> [_ w796]
              tunnel: w794 -> [_ w797]
              frame "About" {
                n361 = call "About.vi"() -> ()  [unwired: 1 out]
              }
              frame Default {
                n362 = Get Menu Item Info(7:w796, 11:w797) -> (2:→"项名称":string)  [unwired: 1 in, 6 out]
              }
            }
          }
          event "返回LOGO": Value Change {
            n363 = event-data() -> ()  [unwired: 2 out]
          }
          event "打开文件夹": Value Change {
            n364 = event-data() -> ()  [unwired: 2 out]
          }
          event "物理参数设置": Value Change {
            n365 = event-data() -> ()  [unwired: 2 out]
          }
          event "多通道并行实测": Value Change {
            n366 = event-data() -> ()  [unwired: 2 out]
            n367 = global write "GlobalVariable.vi" "有无接收"(FALSE ("有无接收")) -> ()
          }
          event "周期拟合与反应性": Value Change {
            n368 = event-data() -> ()  [unwired: 2 out]
          }
        }
        n369 = flat-sequence {
          tunnel: [w786] -> w784
          tunnel: w773 -> [w785]
          tunnel: [w785] -> w783
          frame #0 {
            n370 = global read "GlobalVariable.vi" "有无接收"() -> (w786:bool)
          }
        }
        n371 = Search/Split String ("搜索/拆分字符串")(string=w774, search string/char (-)=":" ("搜索字符串/字符(-)")) -> (substring before match=w781:string)  [unwired: 1 in, 2 out]
        n372 = Equal?(x="仪器设置", y=w781) -> (x = y?=w778:bool)
        n373 = Equal?(x=w781, y="实时测量" ("x")) -> (x = y?=w776:bool)
        n374 = Or(x=w778, y=w776) -> (x .or. y?=w775:bool)
        n375 = case shown="True" w784 {
          tunnel: w783 -> [w787 w789]
          tunnel: [w787 w789] -> w782
          tunnel: w775 -> [_ w788]
          frame False {
          }
          frame True {
            n376 = flat-sequence {
              tunnel: w788 -> [w790]
              frame #0 {
                n377 = global write "GlobalVariable.vi" "返回LOGO"(w790) -> ()
              }
              frame #1 {
                n378 = while {
                  stop <- w791 continue-if-true
                  n379 = global read "GlobalVariable.vi" "返回LOGO"() -> (w791:bool)
                }
              }
            }
          }
        }
      }
    }
    n380 = Equal?(x=w708, y="MainExit") -> (x = y?=w713:bool)
    n381 = Not(x=w713) -> (.not. x?=w716:bool)
    n382 = local read "退出"() -> (w715:bool)
    n383 = Not Equal?(x=w709, y=w708) -> (x != y?=w710:bool)
    n384 = Or(x=w713, y=w715) -> (x .or. y?=w720:bool)
    n385 = And(x=w703, y=w710) -> (x .and. y?=w705:bool)
    n386 = local write "退出"(w720) -> ()
    n387 = And(x=w705, y=w716) -> (x .and. y?=w707:bool)
    n388 = Or(x=w705, y=w713) -> (x .or. y?=w712:bool)
    n389 = case shown="True" w712 {
      tunnel: w718 -> [w724 w727]
      tunnel: [w724 refnum<vi> refnum ("VI Ref")] -> w711
      frame False {
      }
      frame True {
        n390 = invoke class="VI" method="Abort VI"(reference=w727) -> (reference out=w728:refnum<vi>, error out=w729:errorcluster)  [unwired: 2 in, 1 out]
        n391 = Close Reference "关闭引用"(reference=w728, error in (no error)=w729) -> (error out=w725:errorcluster)
        n392 = invoke on="VI_Display" class="SubPnl" method="Remove VI"(error in=w725) -> ()  [unwired: 2 in, 3 out]
      }
    }
    n393 = Not(x=w702) -> (.not. x?=w704:bool)
    n394 = Or(x=w704, y=w707) -> (x .or. y?=w706:bool)
    n395 = case shown="True" w706 {
      tunnel: w711 -> [w735 _]
      tunnel: [w735 w760] -> w723
      tunnel: w708 -> [w731 w756]
      tunnel: [w732 w759] -> w722
      tunnel: w719 -> [w730 w758]
      tunnel: w709 -> [w733 _]
      tunnel: w703 -> [w734 _]
      frame False {
        n396 = case shown="False" w734 {
          tunnel: w733 -> [w750 _]
          tunnel: [w750 w751] -> w732
          tunnel: w731 -> [w739 w751]
          tunnel: w730 -> [w740 _]
          frame False {
            n397 = Build Path(base path=w740, name or relative path=w739) -> (appended path=w738:path)
            n398 = Open VI Reference(type specifier VI Refnum (for type only)=refnum<vi> refnum ("类型说明符VI引用句柄（仅用于类型）"), vi path=w738) -> (vi reference=w746:refnum<vi>, error out=w744:errorcluster)  [unwired: 4 in]
            n399 = invoke class="VI" method="FP.Open"(reference=w746, error in=w744, "Activate"=TRUE ("激活？"), "State"=T2."Standard" ("状态")) -> (reference out=w745:refnum<vi>, error out=w743:errorcluster)  [unwired: 1 in, 3 out]
            n400 = invoke class="VI" method="Run VI"(reference=w745, error in=w743, "Wait until done"=FALSE ("结束前等待"), "Auto Dispose Ref"=TRUE ("自动销毁引用")) -> (reference out=w737:refnum<vi>, error out=w736:errorcluster)  [unwired: 1 in, 3 out]
            n401 = Close Reference(reference=w737, error in (no error)=w736) -> ()  [unwired: 1 out]
          }
          frame True {
          }
        }
      }
      frame True {
        n402 = Equal?(x=w756, y="logo.vi") -> (x = y?=w752:bool)
        n403 = Build Path(base path=w758, name or relative path=w756) -> (appended path=w764:path)
        n404 = call "LoadAndRun.vi"("run?"=TRUE, "path"=w764) -> ("error out"=w761:errorcluster, "vi refnum out"=w762:refnum<vi>)  [unwired: 2 in]
        n405 = Select(t=u32 1, s=w752, f=u32 0) -> (s? t:f=→"MainPanel":u32)
        n406 = case "条件结构" shown="True" w752 {
          tunnel: w756 -> [w768 w769]
          tunnel: w762 -> [w766 w770]
          tunnel: w761 -> [w767 _]
          tunnel: [w766 w770] -> w760
          tunnel: [w768 w769] -> w759
          frame False {
            n407 = invoke on="VI_Display" class="SubPnl" method="Insert VI"(error in=w767, "VI Ref"=w766) -> (error out=w765:errorcluster)  [unwired: 2 in, 3 out]
            n408 = call <vilib>:"Simple Error Handler.vi"("error in (no error)"=w765) -> ()  [unwired: 4 in, 5 out]
          }
          frame True {
          }
        }
      }
    }
    n409 = Wait (ms)(milliseconds to wait=50) -> ()  [unwired: 1 out]
  }
  n410 = case shown="True" w3 {
    frame False {
      w809 = TRUE ("可见")
      n411 = property on="更新物理参数" class="Bool"("Visible"=w809) -> (error out=w810:errorcluster)  [unwired: 2 in, 1 out]
      n412 = property on="离线数据源" class="Bool"(error in=w810, "Visible"=w809) -> ()  [unwired: 1 in, 2 out]
    }
    frame True {
      n413 = invoke class="VI" method="FP.Close"() -> (reference out=w811:refnum<vi>, error out=w812:errorcluster)  [unwired: 3 in, 1 out]
      n414 = Close Reference(reference=w811, error in (no error)=w812) -> ()  [unwired: 1 out]
    }
  }
